vi "Pick Best Target.vi"(1 "Target Infos":T1[](array[typedef])) -> (0 "Best Target Info":T1)   [LabVIEW 2016]
uses:
  Targets Info.ctl
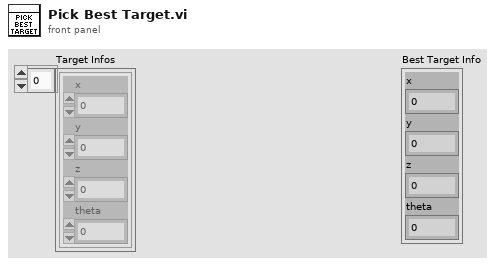
[diagram p1: front panel]
types:
  T1 = typedef "Targets Info.ctl" = cluster{"x":dbl, "y":dbl, "z":dbl, "theta":dbl}
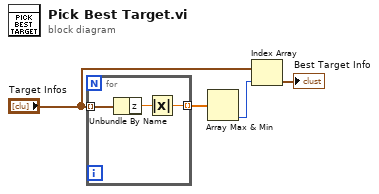
[diagram p0: block diagram]
diagram:
  n1 = for {
    tunnel: "Target Infos" -> [w7] mode=indexing
    tunnel: [w5] -> w4 mode=indexing
    n2 = Unbundle By Name(w7) -> ("z"=w6:dbl)
    n3 = Absolute Value(x=w6) -> (abs(x)=w5:dbl)
  }
  n4 = Array Max & Min(array=w4) -> (min index (indices)=w2:i32)  [unwired: 3 out]
  n5 = Index Array(array="Target Infos", index=w2) -> (element=→"Best Target Info":T1)
